vi "Rectangles to Commands.vi"(5 "Offset":cluster{"X Offset":dbl, "Y Offset":dbl}, 7 "Scaling":T1={"X Scaling (%)"=100.0, "Y Scaling (%)"=100.0}, 8 "error in (no error)":errorcluster, 10 "Rectangle Properties":T3(array[cluster])=[{"Speed"=100.0, "Direction (For Stroked)"=0, "Start Point"=enum."Bottom Left Corner", "Spacing Between Lines\n(For Filled)"=0.02, "Orientation (For Filled)"=enum."Horizontal", "Start and End Voltage"={"End Voltage"=0.0, "Start Voltage"=0.0}}] {"Direction (For Stroked)" items=["Clockwise", "Counterclockwise"]}, 11 "rects":T5(array[cluster])) -> (0 "error out":errorcluster, 3 "Lithography Information":T2(array[cluster]))   [LabVIEW 2011]
doc: "This VI processes the rectangles' data and outputs lithography data."
uses:
  <vilib>/Analysis/Matrix/Datatypes/RealMatrix.ctl
  <vilib>/Analysis/Matrix/NI_Matrix.lvlib
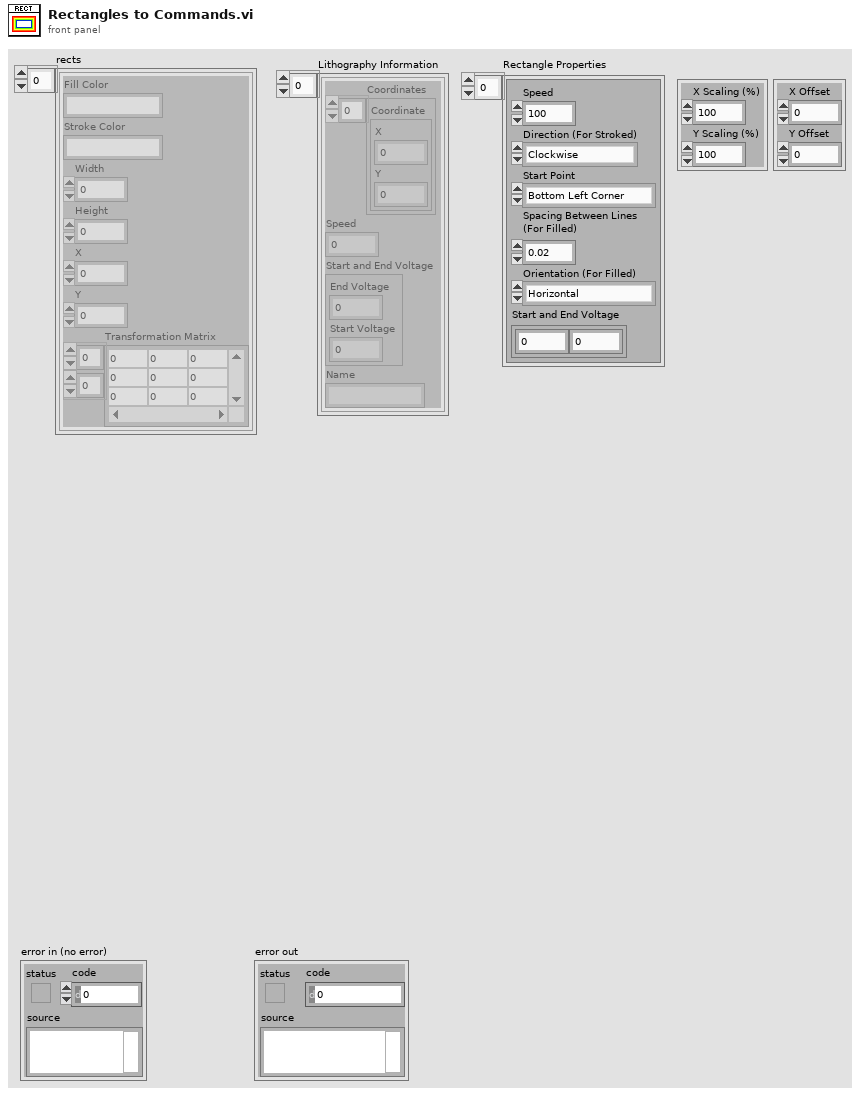
[diagram p1: front panel]
types:
  T1 = cluster{"X Scaling (%)":dbl, "Y Scaling (%)":dbl}
  T2 = cluster{"Coordinates":cluster{"X":dbl, "Y":dbl}[], "Speed":dbl, "Start and End Voltage":cluster{"End Voltage":dbl, "Start Voltage":dbl}, "Name":string}[]
  T3 = cluster{"Speed":dbl, "Direction (For Stroked)":u16, "Start Point":enum16{"Bottom Left Corner", "Bottom Right Corner", "Top Left Corner", "Top Right Corner"}, "Spacing Between Lines\n(For Filled)":dbl, "Orientation (For Filled)":enum16{"Horizontal", "Vertical"}, "Start and End Voltage":cluster{"End Voltage":dbl, "Start Voltage":dbl}}[]
  T4 = typedef "NI_Matrix.lvlib/RealMatrix.ctl" = dbl[][]
  T5 = cluster{"Fill Color":string, "Stroke Color":string, "Width":dbl, "Height":dbl, "X":dbl, "Y":dbl, "Transformation Matrix":T4}[]
  T6 = enum16{"Bottom Left Corner", "Bottom Right Corner", "Top Left Corner", "Top Right Corner"}
  T7 = cluster{cluster{dbl, dbl}[], "Speed":dbl, "Start and End Voltage":cluster{"End Voltage":dbl, "Start Voltage":dbl}, string}
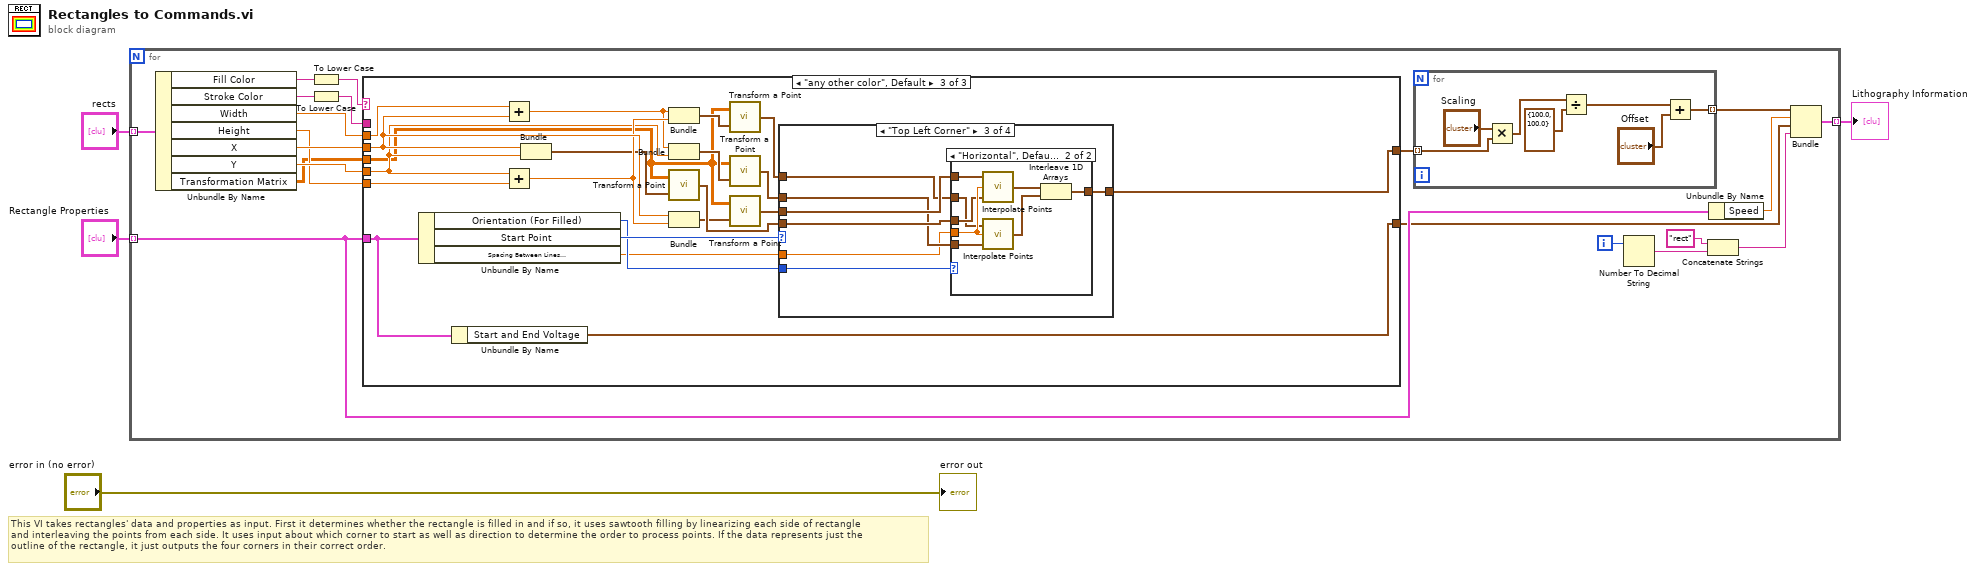
[diagram p0: block diagram]
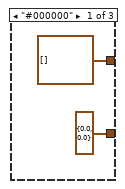
[diagram p2: hidden frame]
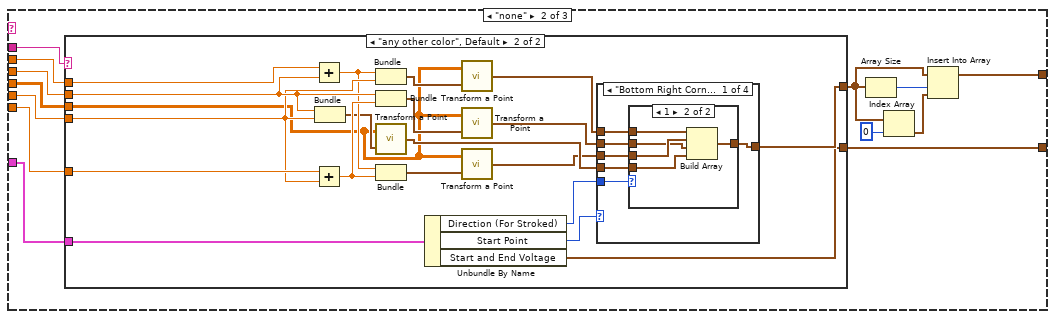
[diagram p3: hidden frame]
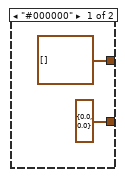
[diagram p4: hidden frame]
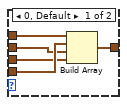
[diagram p5: hidden frame]
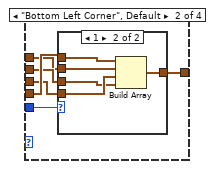
[diagram p6: hidden frame]
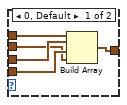
[diagram p7: hidden frame]
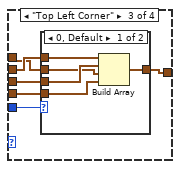
[diagram p8: hidden frame]
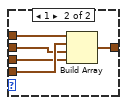
[diagram p9: hidden frame]
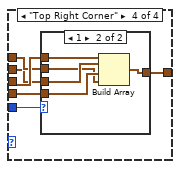
[diagram p10: hidden frame]
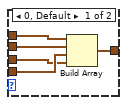
[diagram p11: hidden frame]
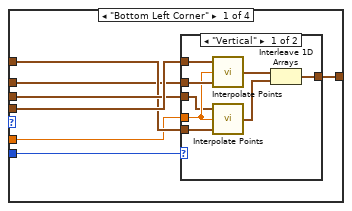
[diagram p12: hidden frame]
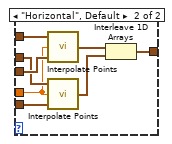
[diagram p13: hidden frame]
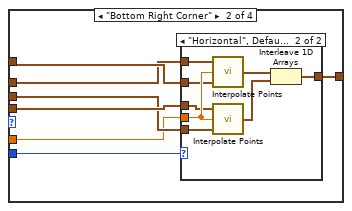
[diagram p14: hidden frame]
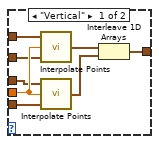
[diagram p15: hidden frame]
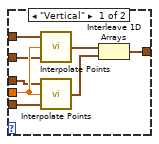
[diagram p16: hidden frame]
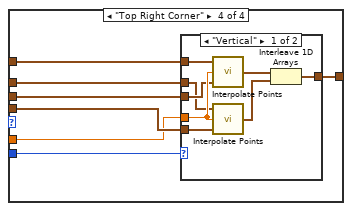
[diagram p17: hidden frame]
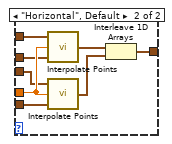
[diagram p18: hidden frame]
diagram:
  # "This VI takes rectangles' data and properties as input. First it determines whether the rectangle is filled in and if so, it uses sawtooth filling by linearizing each side of rectangle \nand interleaving the points from each side. It uses input about which corner to start as well as direction to determine the order to process points. If the data represents just the \noutline of the rectangle, it just outputs the four corners in their correct order."
  n1 = for {
    tunnel: "rects" -> [w24] mode=indexing
    tunnel: "Rectangle Properties" -> [w18] mode=indexing
    tunnel: [w19] -> w1 mode=indexing
    i -> [w14]
    n2 = Unbundle By Name(w24) -> ("Fill Color"=w23:string, "Stroke Color"=w21:string, "Width"=w9:dbl, "Height"=w6:dbl, "X"=w8:dbl, "Y"=w7:dbl, "Transformation Matrix"=w5:T4)
    n3 = To Lower Case(string=w23) -> (all lower case string=w22:string)
    n4 = To Lower Case(string=w21) -> (all lower case string=w20:string)
    n5 = case shown="\"any other color\", Default" w22 {
      tunnel: w20 -> [_ w42 _]
      tunnel: w9 -> [_ w46 w150]
      tunnel: w6 -> [_ w45 w149]
      tunnel: w8 -> [_ w44 w148]
      tunnel: w7 -> [_ w43 w145]
      tunnel: w18 -> [_ w35 w134]
      tunnel: [cluster{"X":dbl, "Y":dbl}[] [] w37 w153] -> w11
      tunnel: w5 -> [_ w36 w135]
      tunnel: [cluster{"End Voltage":dbl, "Start Voltage":dbl} {"End Voltage"=0.0, "Start Voltage"=0.0} ("Start and End Voltage") w34 w133] -> w16
      frame "#000000" {
      }
      frame "none" {
        n6 = case shown="\"any other color\", Default" w42 {
          tunnel: w46 -> [_ w67]
          tunnel: w45 -> [_ w68]
          tunnel: w44 -> [_ w66]
          tunnel: w43 -> [_ w64]
          tunnel: [cluster{"X":dbl, "Y":dbl}[] [] w59] -> w38
          tunnel: w35 -> [_ w62]
          tunnel: w36 -> [_ w50]
          tunnel: [cluster{"End Voltage":dbl, "Start Voltage":dbl} {"End Voltage"=0.0, "Start Voltage"=0.0} ("Start and End Voltage") w49] -> w34
          frame "#000000" {
          }
          frame "any other color", Default {
            n7 = Add(x=w67, y=w66) -> (x+y=w63:dbl)
            n8 = Add(x=w68, y=w64) -> (x+y=w65:dbl)
            n9 = Bundle("X"=w66, "Y"=w64) -> (w56:cluster{"X":dbl, "Y":dbl})  [unwired: 1 in]
            n10 = Bundle(w63, "Y"=w64) -> (w51:cluster{dbl, "Y":dbl})  [unwired: 1 in]
            n11 = Bundle("X"=w66, w65) -> (w58:cluster{"X":dbl, dbl})  [unwired: 1 in]
            n12 = call "Transform a Point.vi"("Point to Transform"=w56, "Transformation Matrix"=w50) -> ("Transformed Point"=w55:cluster{"X":dbl, "Y":dbl})
            n13 = Bundle(w63, w65) -> (w53:cluster{dbl, dbl})  [unwired: 1 in]
            n14 = Unbundle By Name(w62) -> ("Direction (For Stroked)"=w60:u16, "Start Point"=w61:T6, "Start and End Voltage"=w49:cluster{"End Voltage":dbl, "Start Voltage":dbl})
            n15 = call "Transform a Point.vi"("Point to Transform"=w51, "Transformation Matrix"=w50) -> ("Transformed Point"=w52:cluster{"X":dbl, "Y":dbl})
            n16 = call "Transform a Point.vi"("Point to Transform"=w58, "Transformation Matrix"=w50) -> ("Transformed Point"=w57:cluster{"X":dbl, "Y":dbl})
            n17 = call "Transform a Point.vi"("Point to Transform"=w53, "Transformation Matrix"=w50) -> ("Transformed Point"=w54:cluster{"X":dbl, "Y":dbl})
            n18 = case shown="\"Bottom Right Corner\"" w61 {
              tunnel: w60 -> [w74 w90 w106 w122]
              tunnel: [w73 w89 w105 w121] -> w59
              tunnel: w55 -> [w71 w88 w101 w118]
              tunnel: w57 -> [w70 w87 w104 w117]
              tunnel: w54 -> [w69 w86 w103 w120]
              tunnel: w52 -> [w72 w85 w102 w119]
              frame "Bottom Right Corner" {
                n19 = case shown="1" w74 {
                  tunnel: [w79 w84] -> w73
                  tunnel: w72 -> [w78 w83]
                  tunnel: w71 -> [w77 w80]
                  tunnel: w70 -> [w76 w81]
                  tunnel: w69 -> [w75 w82]
                  frame 0, Default {
                    n20 = Build Array(w78, w77, w76, w75) -> (w79:cluster{"X":dbl, "Y":dbl}[])
                  }
                  frame 1 {
                    n21 = Build Array(w83, w82, w81, w80) -> (w84:cluster{"X":dbl, "Y":dbl}[])
                  }
                }
              }
              frame "Bottom Left Corner", Default {
                n22 = case shown="1" w90 {
                  tunnel: [w95 w100] -> w89
                  tunnel: w88 -> [w94 w99]
                  tunnel: w87 -> [w93 w96]
                  tunnel: w86 -> [w92 w97]
                  tunnel: w85 -> [w91 w98]
                  frame 0, Default {
                    n23 = Build Array(w94, w93, w92, w91) -> (w95:cluster{"X":dbl, "Y":dbl}[])
                  }
                  frame 1 {
                    n24 = Build Array(w99, w98, w97, w96) -> (w100:cluster{"X":dbl, "Y":dbl}[])
                  }
                }
              }
              frame "Top Left Corner" {
                n25 = case shown="0, Default" w106 {
                  tunnel: [w111 w116] -> w105
                  tunnel: w104 -> [w110 w115]
                  tunnel: w103 -> [w109 w112]
                  tunnel: w102 -> [w108 w113]
                  tunnel: w101 -> [w107 w114]
                  frame 0, Default {
                    n26 = Build Array(w110, w109, w108, w107) -> (w111:cluster{"X":dbl, "Y":dbl}[])
                  }
                  frame 1 {
                    n27 = Build Array(w115, w114, w113, w112) -> (w116:cluster{"X":dbl, "Y":dbl}[])
                  }
                }
              }
              frame "Top Right Corner" {
                n28 = case shown="1" w122 {
                  tunnel: [w127 w132] -> w121
                  tunnel: w120 -> [w126 w131]
                  tunnel: w119 -> [w125 w128]
                  tunnel: w118 -> [w124 w129]
                  tunnel: w117 -> [w123 w130]
                  frame 0, Default {
                    n29 = Build Array(w126, w125, w124, w123) -> (w127:cluster{"X":dbl, "Y":dbl}[])
                  }
                  frame 1 {
                    n30 = Build Array(w131, w130, w129, w128) -> (w132:cluster{"X":dbl, "Y":dbl}[])
                  }
                }
              }
            }
          }
        }
        n31 = Array Size(array=w38) -> (size(s)=w41:i32)
        n32 = Index Array(array=w38, index=0) -> (element=w40:cluster{"X":dbl, "Y":dbl})
        n33 = Insert Into Array(array=w38, index=w41, new element=w40) -> (w37:cluster{"X":dbl, "Y":dbl}[])
      }
      frame "any other color", Default {
        n34 = Unbundle By Name(w134) -> ("Orientation (For Filled)"=w151:enum16{"Horizontal", "Vertical"}, "Start Point"=w152:T6, "Spacing Between Lines\n(For Filled)"=w144:dbl)
        n35 = Unbundle By Name(w134) -> ("Start and End Voltage"=w133:cluster{"End Voltage":dbl, "Start Voltage":dbl})
        n36 = Add(x=w150, y=w148) -> (x+y=w146:dbl)
        n37 = Add(x=w145, y=w149) -> (x+y=w147:dbl)
        n38 = Bundle("X"=w148, "Y"=w145) -> (w143:cluster{"X":dbl, "Y":dbl})  [unwired: 1 in]
        n39 = Bundle(w146, w147) -> (w141:cluster{dbl, dbl})  [unwired: 1 in]
        n40 = Bundle(w146, "Y"=w145) -> (w136:cluster{dbl, "Y":dbl})  [unwired: 1 in]
        n41 = call "Transform a Point.vi"("Point to Transform"=w143, "Transformation Matrix"=w135) -> ("Transformed Point"=w142:cluster{"X":dbl, "Y":dbl})
        n42 = Bundle("X"=w148, w147) -> (w139:cluster{"X":dbl, dbl})  [unwired: 1 in]
        n43 = call "Transform a Point.vi"("Point to Transform"=w141, "Transformation Matrix"=w135) -> ("Transformed Point"=w140:cluster{"X":dbl, "Y":dbl})
        n44 = call "Transform a Point.vi"("Point to Transform"=w136, "Transformation Matrix"=w135) -> ("Transformed Point"=w137:cluster{"X":dbl, "Y":dbl})
        n45 = call "Transform a Point.vi"("Point to Transform"=w139, "Transformation Matrix"=w135) -> ("Transformed Point"=w138:cluster{"X":dbl, "Y":dbl})
        n46 = case shown="\"Top Left Corner\"" w152 {
          tunnel: w151 -> [w160 w183 w206 w229]
          tunnel: [w159 w182 w205 w228] -> w153
          tunnel: w137 -> [w155 w178 w201 w224]
          tunnel: w140 -> [w156 w179 w202 w225]
          tunnel: w138 -> [w157 w180 w203 w226]
          tunnel: w142 -> [w158 w181 w204 w227]
          tunnel: w144 -> [w154 w177 w200 w223]
          frame "Bottom Left Corner" {
            n47 = case shown="\"Vertical\"" w160 {
              tunnel: [w166 w176] -> w159
              tunnel: w158 -> [w165 w175]
              tunnel: w157 -> [w162 w174]
              tunnel: w156 -> [w161 w172]
              tunnel: w155 -> [w164 w173]
              tunnel: w154 -> [w163 w171]
              frame "Vertical" {
                n48 = call "Interpolate Points.vi"("End Point"=w164, "Distance between Points"=w163, "Start Point"=w165) -> ("Output Point Array"=w168:cluster{"X":dbl, "Y":dbl}[])
                n49 = call "Interpolate Points.vi"("End Point"=w161, "Distance between Points"=w163, "Start Point"=w162) -> ("Output Point Array"=w167:cluster{"X":dbl, "Y":dbl}[])
                n50 = Interleave 1D Arrays(w168, w167) -> (w166:cluster{"X":dbl, "Y":dbl}[])
              }
              frame "Horizontal", Default {
                n51 = call "Interpolate Points.vi"("End Point"=w174, "Distance between Points"=w171, "Start Point"=w175) -> ("Output Point Array"=w170:cluster{"X":dbl, "Y":dbl}[])
                n52 = call "Interpolate Points.vi"("End Point"=w172, "Distance between Points"=w171, "Start Point"=w173) -> ("Output Point Array"=w169:cluster{"X":dbl, "Y":dbl}[])
                n53 = Interleave 1D Arrays(w170, w169) -> (w176:cluster{"X":dbl, "Y":dbl}[])
              }
            }
          }
          frame "Bottom Right Corner" {
            n54 = case shown="\"Horizontal\", Default" w183 {
              tunnel: [w189 w199] -> w182
              tunnel: w181 -> [w185 w193]
              tunnel: w180 -> [w184 w192]
              tunnel: w179 -> [w186 w194]
              tunnel: w178 -> [w187 w195]
              tunnel: w177 -> [w188 w198]
              frame "Vertical" {
                n55 = call "Interpolate Points.vi"("End Point"=w186, "Distance between Points"=w188, "Start Point"=w187) -> ("Output Point Array"=w191:cluster{"X":dbl, "Y":dbl}[])
                n56 = call "Interpolate Points.vi"("End Point"=w184, "Distance between Points"=w188, "Start Point"=w185) -> ("Output Point Array"=w190:cluster{"X":dbl, "Y":dbl}[])
                n57 = Interleave 1D Arrays(w191, w190) -> (w189:cluster{"X":dbl, "Y":dbl}[])
              }
              frame "Horizontal", Default {
                n58 = call "Interpolate Points.vi"("End Point"=w194, "Distance between Points"=w198, "Start Point"=w195) -> ("Output Point Array"=w197:cluster{"X":dbl, "Y":dbl}[])
                n59 = call "Interpolate Points.vi"("End Point"=w192, "Distance between Points"=w198, "Start Point"=w193) -> ("Output Point Array"=w196:cluster{"X":dbl, "Y":dbl}[])
                n60 = Interleave 1D Arrays(w197, w196) -> (w199:cluster{"X":dbl, "Y":dbl}[])
              }
            }
          }
          frame "Top Left Corner" {
            n61 = case shown="\"Horizontal\", Default" w206 {
              tunnel: [w212 w222] -> w205
              tunnel: w204 -> [w208 w217]
              tunnel: w203 -> [w210 w218]
              tunnel: w202 -> [w209 w216]
              tunnel: w201 -> [w207 w215]
              tunnel: w200 -> [w211 w221]
              frame "Vertical" {
                n62 = call "Interpolate Points.vi"("End Point"=w209, "Distance between Points"=w211, "Start Point"=w210) -> ("Output Point Array"=w214:cluster{"X":dbl, "Y":dbl}[])
                n63 = call "Interpolate Points.vi"("End Point"=w207, "Distance between Points"=w211, "Start Point"=w208) -> ("Output Point Array"=w213:cluster{"X":dbl, "Y":dbl}[])
                n64 = Interleave 1D Arrays(w214, w213) -> (w212:cluster{"X":dbl, "Y":dbl}[])
              }
              frame "Horizontal", Default {
                n65 = call "Interpolate Points.vi"("End Point"=w217, "Distance between Points"=w221, "Start Point"=w218) -> ("Output Point Array"=w220:cluster{"X":dbl, "Y":dbl}[])
                n66 = call "Interpolate Points.vi"("End Point"=w215, "Distance between Points"=w221, "Start Point"=w216) -> ("Output Point Array"=w219:cluster{"X":dbl, "Y":dbl}[])
                n67 = Interleave 1D Arrays(w220, w219) -> (w222:cluster{"X":dbl, "Y":dbl}[])
              }
            }
          }
          frame "Top Right Corner" {
            n68 = case shown="\"Vertical\"" w229 {
              tunnel: [w235 w245] -> w228
              tunnel: w227 -> [w230 w238]
              tunnel: w226 -> [w232 w239]
              tunnel: w225 -> [w233 w241]
              tunnel: w224 -> [w231 w240]
              tunnel: w223 -> [w234 w244]
              frame "Vertical" {
                n69 = call "Interpolate Points.vi"("End Point"=w232, "Distance between Points"=w234, "Start Point"=w233) -> ("Output Point Array"=w237:cluster{"X":dbl, "Y":dbl}[])
                n70 = call "Interpolate Points.vi"("End Point"=w230, "Distance between Points"=w234, "Start Point"=w231) -> ("Output Point Array"=w236:cluster{"X":dbl, "Y":dbl}[])
                n71 = Interleave 1D Arrays(w237, w236) -> (w235:cluster{"X":dbl, "Y":dbl}[])
              }
              frame "Horizontal", Default {
                n72 = call "Interpolate Points.vi"("End Point"=w240, "Distance between Points"=w244, "Start Point"=w241) -> ("Output Point Array"=w243:cluster{"X":dbl, "Y":dbl}[])
                n73 = call "Interpolate Points.vi"("End Point"=w238, "Distance between Points"=w244, "Start Point"=w239) -> ("Output Point Array"=w242:cluster{"X":dbl, "Y":dbl}[])
                n74 = Interleave 1D Arrays(w243, w242) -> (w245:cluster{"X":dbl, "Y":dbl}[])
              }
            }
          }
        }
      }
    }
    n75 = for {
      tunnel: w11 -> [w31] mode=indexing
      tunnel: [w26] -> w10 mode=indexing
      n76 = Multiply(x="Scaling", y=w31) -> (x*y=w29:cluster{dbl, dbl})
      n77 = Divide(x=w29, y=cluster{dbl, dbl} {100.0, 100.0}) -> (x/y=w27:cluster{dbl, dbl})
      n78 = Add(x=w27, y="Offset") -> (x+y=w26:cluster{dbl, dbl})
    }
    n79 = Number To Decimal String(number=w14) -> (decimal integer string=w13:string)  [unwired: 1 in]
    n80 = Concatenate Strings("rect", w13) -> (w12:string)
    n81 = Unbundle By Name(w18) -> ("Speed"=w17:dbl)
    n82 = Bundle(w10, "Speed"=w17, "Start and End Voltage"=w16, w12) -> (w19:T7)  [unwired: 1 in]
  }
  "Lithography Information" <- w1
  "error out" <- "error in (no error)"
